vi "List Neighbours.vi"(0 "Cell Index":i32, 11 "error in (no error)":errorcluster) -> (4 "Neighbours":i32[](array[numeric]), 6 "Max Capacity":i32, 15 "error out":errorcluster)   [LabVIEW 2014, in "Dragon Tamers.lvlib"]
uses:
  Dragon Tamers.lvlib
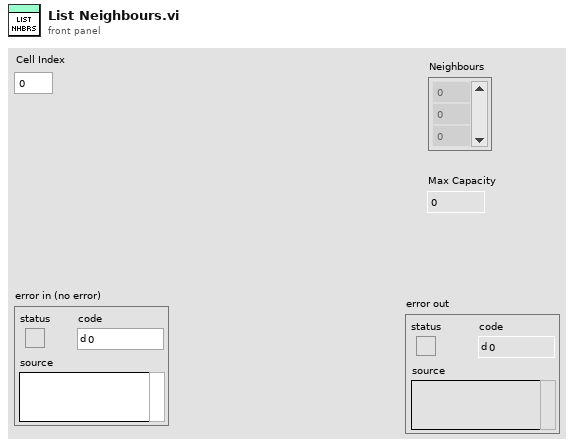
[diagram p1: front panel]
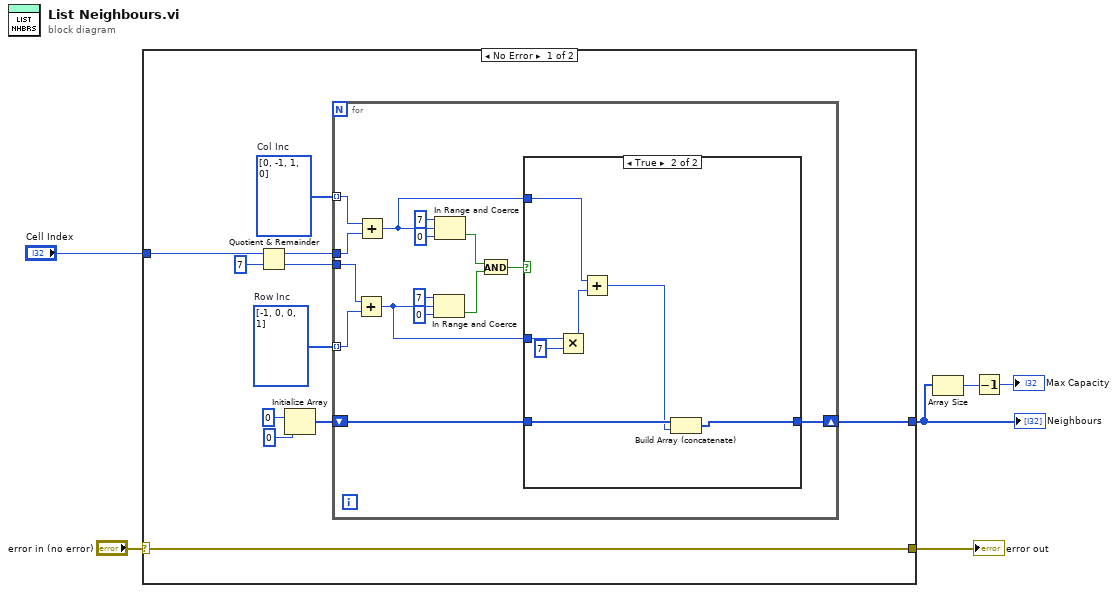
[diagram p0: block diagram]
diagram:
  n1 = case shown="No Error" "error in (no error)" {
    selector: "error in (no error)" -> [w8 w41]
    tunnel: [w8 w41] -> w5
    tunnel: "Cell Index" -> [w17 _]
    tunnel: [w7 _] -> w3
    frame No Error {
      w10 = i32[] [0, -1, 1, 0]  # Col Inc
      w9 = i32[] [-1, 0, 0, 1]  # Row Inc
      n2 = Quotient & Remainder(x=w17, y=7) -> (x-y*floor(x/y)=w15:i32, floor(x/y)=w14:i32)
      n3 = Initialize Array(0, 0 ("dimension size")) -> (w13:i32[])
      n4 = for {
        tunnel: w15 -> [w29]
        tunnel: w14 -> [w32]
        shift-right: [w18] -> w7
        shift-left: w13 -> [w19]
        tunnel: w10 -> [w30] mode=indexing
        tunnel: w9 -> [w31] mode=indexing
        n5 = Add(x=w32, y=w31) -> (x+y=w20:i32)
        n6 = Add(x=w30, y=w29) -> (x+y=w21:i32)
        n7 = In Range and Coerce(upper limit=7, x=w20, lower limit=0) -> (In Range?=w23:bool)  [unwired: 1 out]
        n8 = In Range and Coerce(upper limit=7, x=w21, lower limit=0) -> (In Range?=w24:bool)  [unwired: 1 out]
        n9 = And(x=w24, y=w23) -> (x .and. y?=w22:bool)
        n10 = case shown="True" w22 {
          tunnel: w21 -> [_ w37]
          tunnel: w20 -> [_ w40]
          tunnel: w19 -> [w33 w36]
          tunnel: [w33 w34] -> w18
          frame False {
          }
          frame True {
            n11 = Multiply(x=w40, y=7) -> (x*y=w38:i32)
            n12 = Add(x=w37, y=w38) -> (x+y=w35:i32)
            n13 = Build Array (concatenate)(w36, w35) -> (w34:i32[])
          }
        }
      }
    }
    frame Error {
    }
  }
  "error out" <- w5
  "Neighbours" <- w3
  n14 = Array Size(array=w3) -> (size(s)=w2:i32)
  n15 = Decrement(x=w2) -> (x-1=→"Max Capacity":i32)
